vi "DebugTool.vi"(8 "Fehler (Eingang, kein Fehler)":errorcluster, 10 "String":string, 11 "Numerisch":dbl format="%#_13g") -> (0 "error out":errorcluster caption="Fehler (Ausgang)")   [LabVIEW 2013]
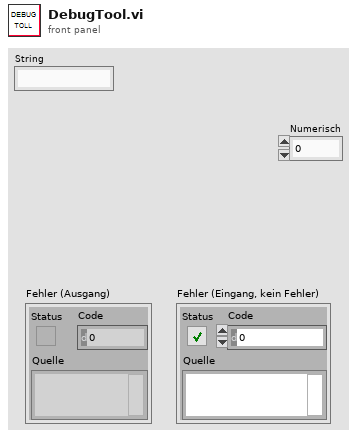
[diagram p1: front panel]
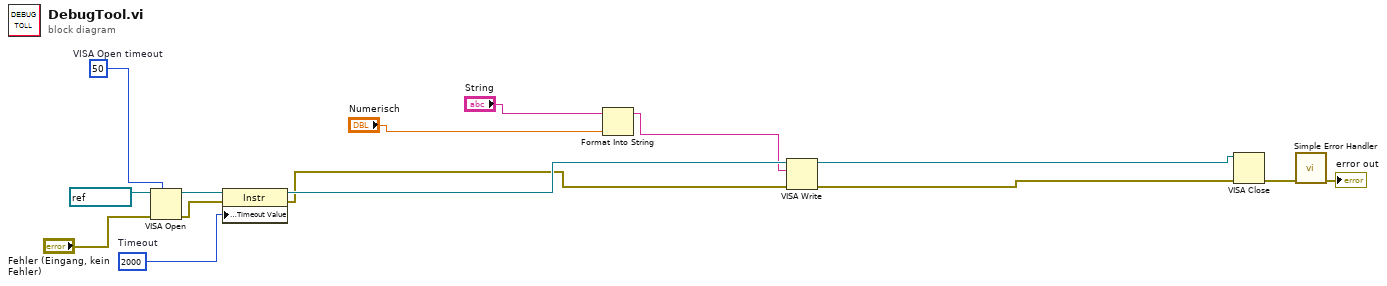
[diagram p0: block diagram]
diagram:
  w10 = u32 50  # VISA Open timeout
  w12 = u32 2000  # Timeout
  n1 = VISA Open(timeout (0)=w10, error in (no error)="Fehler (Eingang, kein Fehler)", VISA resource name=refnum<visa-resource-name> "COM1" ("VISA-Ressourcenname")) -> (VISA resource name=w13:refnum<visa-resource-name>, error out=w14:errorcluster)  [unwired: 2 in]
  n2 = property class="Instr"(reference=w13, error in=w14, "General Settings:Timeout Value"=w12) -> (reference out=w11:refnum<visa-resource-name>, error out=w9:errorcluster)
  n3 = Format Into String(initial string="String", "Numerisch") -> (resulting string=w3:string)  [unwired: 2 in, 1 out]
  n4 = VISA Write(VISA resource name=w11, write buffer=w3, error in (no error)=w9) -> (VISA resource name out=w7:refnum<visa-resource-name>, error out=w6:errorcluster)  [unwired: 1 out]
  n5 = VISA Close(VISA resource name=w7, error in (no error)=w6) -> (error out=w8:errorcluster)
  n6 = call <vilib>:"Simple Error Handler.vi"("error in (no error)"=w8) -> ("error out"=→"error out":errorcluster)  [unwired: 4 in, 4 out]
